vi "Get Pixel - High Speed (SubVI).vi"(9 "Dim":u32=256, 10 "Colum In":u32, 11 "Current A pixel base (row) in":u32) -> (1 "Pixel B":u32, 2 "Pixel A":u32, 3 "Current A pixel base (row) out":u32)   [LabVIEW 2017]
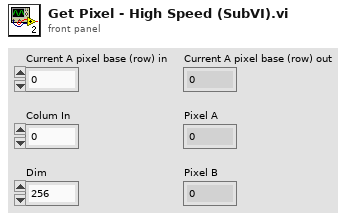
[diagram p1: front panel]
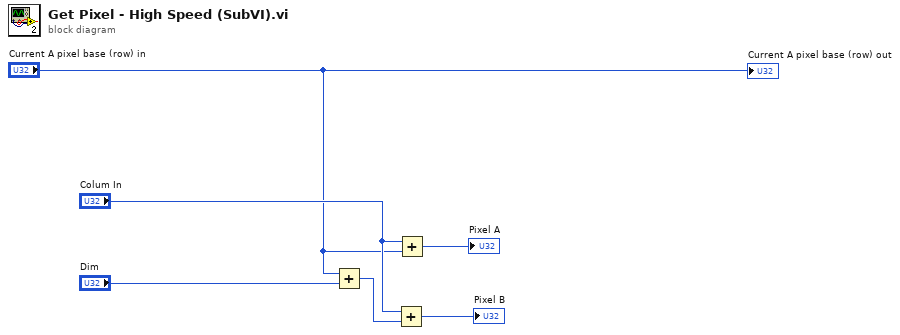
[diagram p0: block diagram]
diagram:
  n1 = Add(x="Current A pixel base (row) in", y="Dim") -> (x+y=w5:u32)
  n2 = Add(x="Colum In", y=w5) -> (x+y=→"Pixel B":u32)
  n3 = Add(x="Colum In", y="Current A pixel base (row) in") -> (x+y=→"Pixel A":u32)
  "Current A pixel base (row) out" <- "Current A pixel base (row) in"
